vi "ConvertC-F.vi"(3 "Tolerance":dbl, 5 "Distance(mA.)":dbl) -> (0 "LowerForce(N.)":dbl format="%#_13g", 1 "NormalForce(N.)":dbl, 2 "UpperForce(N.)":dbl format="%#_13g")   [LabVIEW 2017]
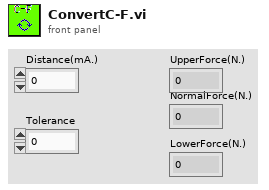
[diagram p1: front panel]
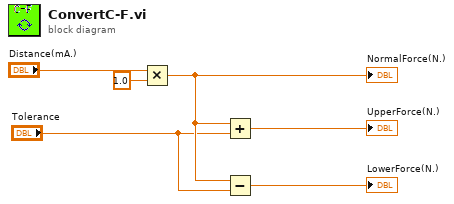
[diagram p0: block diagram]
diagram:
  n1 = Multiply(x="Distance(mA.)", y=1.0) -> (x*y=w2:dbl)
  "NormalForce(N.)" <- w2
  n2 = Add(x=w2, y="Tolerance") -> (x+y=→"UpperForce(N.)":dbl)
  n3 = Subtract(x=w2, y="Tolerance") -> (x-y=→"LowerForce(N.)":dbl)
